vi "Save_enable.vi"(8 "error in (no error)":errorcluster, 10 "Save":bool, 11 "Contador_Bin_Actor in":refnum<class "Contador_Bin_Actor.lvclass">) -> (0 "error out":errorcluster, 3 "Contador_Bin_Actor out":refnum<class "Contador_Bin_Actor.lvclass">)   [LabVIEW 2019, in "Contador_Bin_Actor.lvlib" / "Contador_Bin_Actor.lvclass"]
uses:
  Contador_Bin_Actor.lvclass
  Contador_Bin_Actor.lvclass/Contador_Bin_Actor.ctl
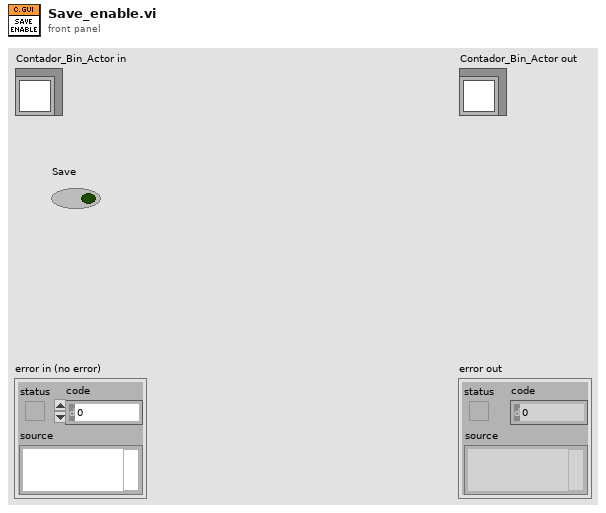
[diagram p1: front panel]
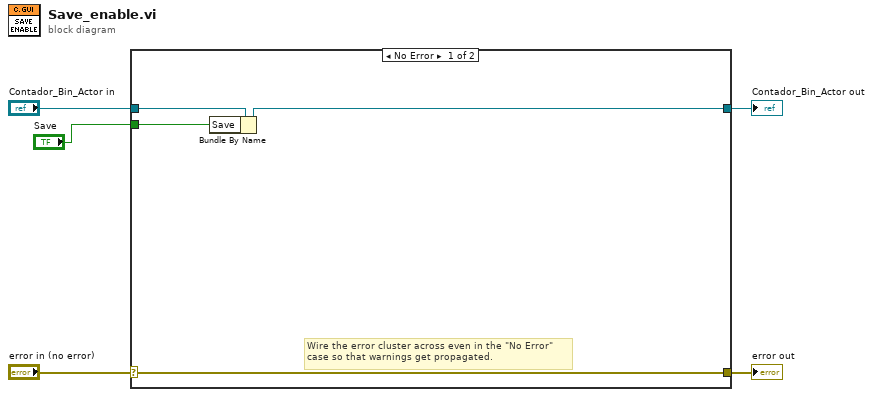
[diagram p0: block diagram]
diagram:
  n1 = case shown="No Error" "error in (no error)" {
    selector: "error in (no error)" -> [w8 w11]
    tunnel: [w8 w11] -> w4
    tunnel: [w7 w10] -> w2
    tunnel: "Contador_Bin_Actor in" -> [w9 w10]
    tunnel: "Save" -> [w6 _]
    frame No Error {
      # "Wire the error cluster across even in the \"No Error\"\ncase so that warnings get propagated."
      n2 = Bundle By Name(cluster=w9, "Save"=w6) -> (w7:refnum<class "Contador_Bin_Actor.lvclass">)
    }
    frame Error {
    }
  }
  "error out" <- w4
  "Contador_Bin_Actor out" <- w2
